vi "保存配置表格.vi"(11 "配置表格":string[][](array[string])) -> ()   [LabVIEW 2016, in "数据传输系统-04.lvlib"]
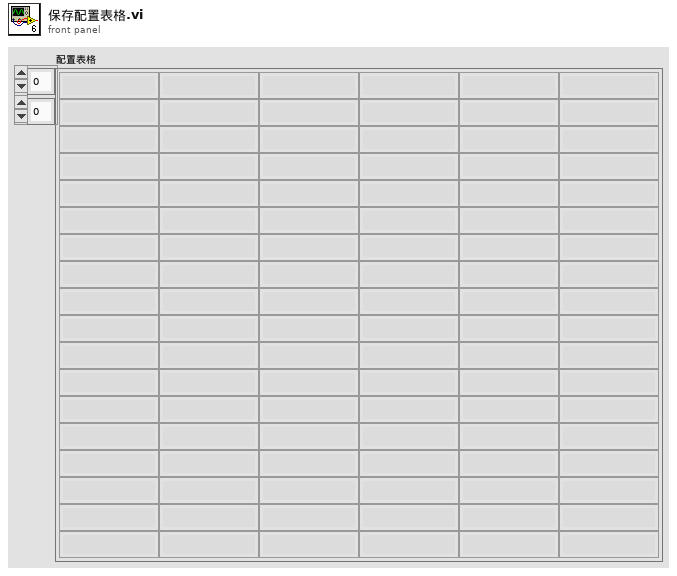
[diagram p1: front panel]
types:
  T1 = cluster{"配置表格[0]":string, "配置表格[1]":string, "配置表格[2]":string, "配置表格[3]":string, "配置表格[4]":string, "配置表格[5]":string, "配置表格[6]":string, "配置表格[7]":string, "配置表格[8]":string, "配置表格[9]":string, "配置表格[10]":string, "配置表格[11]":string, "配置表格[12]":string, "配置表格[13]":string, "配置表格[14]":string, "配置表格[15]":string, "配置表格[16]":string, "配置表格[17]":string, "配置表格[18]":string, "配置表格[19]":string, "配置表格[20]":string, "配置表格[21]":string, "配置表格[22]":string, "配置表格[23]":string, "配置表格[24]":string, "配置表格[25]":string, "配置表格[26]":string, "配置表格[27]":string, "配置表格[28]":string, "配置表格[29]":string, "配置表格[30]":string, "配置表格[31]":string, "配置表格[32]":string, "配置表格[33]":string, "配置表格[34]":string, "配置表格[35]":string, "配置表格[36]":string, "配置表格[37]":string, "配置表格[38]":string, "配置表格[39]":string, "配置表格[40]":string, "配置表格[41]":string, "配置表格[42]":string, "配置表格[43]":string, "配置表格[44]":string, "配置表格[45]":string, "配置表格[46]":string, "配置表格[47]":string, "配置表格[48]":string, "配置表格[49]":string, "配置表格[50]":string, "配置表格[51]":string, "配置表格[52]":string, "配置表格[53]":string, "配置表格[54]":string, "配置表格[55]":string, "配置表格[56]":string, "配置表格[57]":string, "配置表格[58]":string, "配置表格[59]":string, "配置表格[60]":string, "配置表格[61]":string, "配置表格[62]":string, "配置表格[63]":string, "配置表格[64]":string, "配置表格[65]":string, "配置表格[66]":string, "配置表格[67]":string, "配置表格[68]":string, "配置表格[69]":string, "配置表格[70]":string, "配置表格[71]":string, "配置表格[72]":string, "配置表格[73]":string, "配置表格[74]":string, "配置表格[75]":string}
  T2 = cluster{"[0]":dbl, "[1]":dbl, "[2]":dbl, "[3]":dbl, "[4]":dbl, "[5]":dbl, "[6]":dbl, "[7]":dbl, "[8]":dbl, "[9]":dbl, "[10]":dbl, "[11]":dbl, "[12]":dbl, "[13]":dbl, "[14]":dbl, "[15]":dbl, "[16]":dbl, "[17]":dbl, "[18]":dbl, "[19]":dbl, "[20]":dbl, "[21]":dbl, "[22]":dbl, "[23]":dbl, "[24]":dbl, "[25]":dbl, "[26]":dbl, "[27]":dbl, "[28]":dbl, "[29]":dbl, "[30]":dbl, "[31]":dbl, "[32]":dbl, "[33]":dbl, "[34]":dbl, "[35]":dbl, "[36]":dbl, "[37]":dbl, "[38]":dbl, "[39]":dbl, "[40]":dbl, "[41]":dbl, "[42]":dbl, "[43]":dbl, "[44]":dbl, "[45]":dbl, "[46]":dbl, "[47]":dbl, "[48]":dbl, "[49]":dbl, "[50]":dbl, "[51]":dbl, "[52]":dbl, "[53]":dbl, "[54]":dbl, "[55]":dbl, "[56]":dbl, "[57]":dbl, "[58]":dbl, "[59]":dbl, "[60]":dbl, "[61]":dbl, "[62]":dbl, "[63]":dbl, "[64]":dbl, "[65]":dbl, "[66]":dbl, "[67]":dbl, "[68]":dbl, "[69]":dbl, "[70]":dbl, "[71]":dbl, "[72]":dbl, "[73]":dbl, "[74]":dbl, "[75]":dbl}
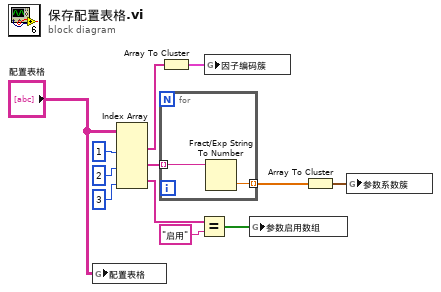
[diagram p0: block diagram]
diagram:
  n1 = global write "断电保存全局.vi" "配置表格"("配置表格") -> ()
  n2 = Index Array(array="配置表格", index (col) #1=1 ("索引 (列)"), index (col) #2=2 ("索引 (列)"), index (col) #3=3 ("索引 (列)")) -> (element #1=w5:string[], element #2=w8:string[], element #3=w9:string[])  [unwired: 3 in]
  n3 = for {
    tunnel: w8 -> [w14] mode=indexing
    tunnel: [w13] -> w7 mode=indexing
    n4 = Fract/Exp String To Number(string=w14) -> (number=w13:dbl)  [unwired: 3 in, 1 out]
  }
  n5 = Array To Cluster(array=w5) -> (cluster=w4:T1)
  n6 = Equal?(x=w9, y="启用") -> (x = y?=w2:bool[])
  n7 = global write "断电保存全局.vi" "因子编码簇"(w4) -> ()
  n8 = global write "断电保存全局.vi" "参数启用数组"(w2) -> ()
  n9 = Array To Cluster(array=w7) -> (cluster=w6:T2)
  n10 = global write "断电保存全局.vi" "参数系数簇"(w6) -> ()
